vi "Ex 05 - Multiple Channels.vi"() -> ()   [LabVIEW 2026]
uses:
  Public/Data/Datatypes/MP - multi-gate inspection.ctl
  Public/Data/Datatypes/MP - multigate inspection gate parameters.ctl
  Public/Data/Datatypes/MP - hysteresis level.ctl
  Public/Data/Datatypes/MP - multigate mode.ctl
  Public/Data/Datatypes/MP - echo gate parameters.ctl
  Public/Data/Datatypes/MP - echo gate mode.ctl
  Public/Data/Datatypes/MP - data formatting.ctl
  Public/Data/Datatypes/MP - amplitude reporting mode.ctl
  Public/Data/Datatypes/MP - averaging.ctl
  Public/Data/Datatypes/MP - transmit parameters.ctl
  Public/Data/Datatypes/MP - pulser voltage.ctl
  Public/Data/Datatypes/MP - pulse damping.ctl
  Public/Data/Datatypes/MP - test parameters.ctl
  Public/Data/Datatypes/MP - receive parameters.ctl
  Public/Data/Datatypes/MP - display gate.ctl
  Public/Data/Datatypes/MP - waveform type.ctl
  Public/Data/Datatypes/MP - analogue filter.ctl
  Public/Data/Datatypes/MP - frequency filter.ctl
  Public/Data/Datatypes/MP - digital filtering.ctl
  Public/Data/Datatypes/MP - high pass filter.ctl
  Public/Data/Datatypes/MP - low pass filter.ctl
  Public/Data/Datatypes/TCP config.ctl
  Public/Data/Datatypes/MP - data output format.ctl
  Public/Data/Datatypes/MP - sample frequency.ctl
  Public/Data/Datatypes/MP - instrument type.ctl
  SubVIs/Main Program State - Enum.ctl
  <vilib>/ErrorRing/Error Ring.xnode
  MicroPulse_Driver.lvlib
panel:
  out "Instrument Type":T1
  out "Sample Frequency out":T2 caption="Sample Frequency"
  out "Stop":bool
  in  "Sample Frequency":T2
  in  "PRF":u16=500 caption="[PRF]" min=1 max=20000 step=100 format="%dHz"
  in  "Data Output Format":T3=enum."8-bit Mode" caption="[DOF]"
  in  "Gate No. 2":i32=1
  out "peak data 2":cluster{"Time":dbl[], "Level":u16[]} {"Time" format="%_6g"}
  out "A-Scan + Peaks 2":cluster{"timebase":dbl[], "data":u16[]}[](graph) caption="A-Scan + Peaks Test 2"
  out "running average PRF 2":dbl format="%0.2f"
  out "live error out 2":errorcluster
  in  "Channel Tab":enum32{"Test 1", "Test 2"}(tab)
  in  "Test 1 Tab":enum32{"Ultrasonic Parameters", "Gates"}(tab)
  in  "Data Formatting":T4={"Amplitude Mode"=enum."Peaks + Ascan for Multigate", "Averaging"=enum."None", "Coupling Level"=0} {"Coupling Level" max=4095 step=1}
  in  "Transmit Parameters":T7={"Pulse Voltage"=enum."50V", "Pulse Shape"={"Damping"=enum."660W", "Width"=250}} {"Pulse Shape"."Width" min=16 max=1010 step=50 format="%.0fns"}
  in  "Test Parameters":T10={"Test No."=1, "Tx Channel"=1, "Rx Channel"=1} {"Rx Channel" min=1 max=1024; "Tx Channel" min=1 max=1024}
  in  "Receive Parameters":T11={"Display Gate"={"Start"=0.0, "Length"=100.0}, "Delay"=0.0, "Waveform Type"=enum."Rectified Signal", "Gain"=50.0, "Analogue Filtering"={"Bandpass"=enum."No change", "Smoothing"=1}, "Digital Filtering"={"High Pass Filter"=enum."None", "Low Pass Filter"=enum."None"}} {"Delay" format="%#_g us"; "Display Gate"."Length" min=0.0 max=64000.0 step=1.0 format="%#_g us"; "Display Gate"."Start" min=0.0 max=64000.0 step=1.0 format="%#_g us"; "Analogue Filtering"."Smoothing" min=1 max=11 step=1; "Gain" min=-6.0 max=70.0 step=0.25 format="%.2fdB"}
  in  "Multi Gate Inspection":T19={"Gate 1"={"Start (us)"=15.0, "Length (us)"=10.0, "Threshold"=80, "Enabled?"=TRUE, "Max # Peaks"=8, "Hysteresis"=enum."6dB", "Mode"=enum."All Peaks In Gate", "Inverted?"=FALSE, "Colour "=16716306}, "Gate 2"={"Start (us)"=30.0, "Length (us)"=10.0, "Threshold"=50, "Enabled?"=TRUE, "Max # Peaks"=8, "Hysteresis"=enum."6dB", "Mode"=enum."All Peaks In Gate", "Inverted?"=FALSE, "Colour "=641024}, "Gate 3"={"Start (us)"=50.0, "Length (us)"=10.0, "Threshold"=30, "Enabled?"=TRUE, "Max # Peaks"=8, "Hysteresis"=enum."6dB", "Mode"=enum."All Peaks In Gate", "Inverted?"=FALSE, "Colour "=4532}, "Gate 4"={"Start (us)"=65.0, "Length (us)"=10.0, "Threshold"=10, "Enabled?"=TRUE, "Max # Peaks"=8, "Hysteresis"=enum."6dB", "Mode"=enum."All Peaks In Gate", "Inverted?"=FALSE, "Colour "=8978537}} {"Gate 4"."Max # Peaks" min=1 max=80 step=1; "Gate 4"."Threshold" min=10 step=10; "Gate 4"."Length (us)" min=0.0 max=96000.0 step=1.0; "Gate 4"."Start (us)" min=0.0 max=64000.0 step=1.0; "Gate 3"."Max # Peaks" min=1 max=80 step=1; "Gate 3"."Threshold" min=10 step=10; "Gate 3"."Length (us)" min=0.0 max=96000.0 step=1.0; "Gate 3"."Start (us)" min=0.0 max=64000.0 step=1.0; "Gate 2"."Max # Peaks" min=1 max=80 step=1; "Gate 2"."Threshold" min=10 step=10; "Gate 2"."Length (us)" min=0.0 max=96000.0 step=1.0; "Gate 2"."Start (us)" min=0.0 max=64000.0 step=1.0; "Gate 1"."Max # Peaks" min=1 max=80 step=1; "Gate 1"."Threshold" min=10 step=10; "Gate 1"."Length (us)" min=0.0 max=96000.0 step=1.0; "Gate 1"."Start (us)" min=0.0 max=64000.0 step=1.0}
  in  "Echo Gate Parameters":T23={"Start (us)"=15.0, "Length (us)"=20.0, "Threshold"=10, "Colour"=2731480} {"Threshold" min=10 max=4095 step=10; "Length (us)" min=0.0 max=96000.0 step=1.0; "Start (us)" min=0.0 max=64000.0 step=1.0}
  in  "Echo Gate Mode":T24
  in  "Test 1 Tab 2":enum32{"Ultrasonic Parameters", "Gates"}(tab)
  in  "Data Formatting 2":T4={"Amplitude Mode"=enum."Peaks + Ascan for Multigate", "Averaging"=enum."None", "Coupling Level"=0} {"Coupling Level" max=4095 step=1}
  in  "Transmit Parameters 2":T7={"Pulse Voltage"=enum."50V", "Pulse Shape"={"Damping"=enum."660W", "Width"=250}} {"Pulse Shape"."Width" min=16 max=1010 step=50 format="%.0fns"}
  in  "Test Parameters 2":T10={"Test No."=1, "Tx Channel"=2, "Rx Channel"=2} {"Rx Channel" min=1 max=1024; "Tx Channel" min=1 max=1024}
  in  "Receive Parameters 2":T11={"Display Gate"={"Start"=0.0, "Length"=100.0}, "Delay"=0.0, "Waveform Type"=enum."Rectified Signal", "Gain"=50.0, "Analogue Filtering"={"Bandpass"=enum."No change", "Smoothing"=1}, "Digital Filtering"={"High Pass Filter"=enum."None", "Low Pass Filter"=enum."None"}} {"Delay" format="%#_g us"; "Display Gate"."Length" min=0.0 max=64000.0 step=1.0 format="%#_g us"; "Display Gate"."Start" min=0.0 max=64000.0 step=1.0 format="%#_g us"; "Analogue Filtering"."Smoothing" min=1 max=11 step=1; "Gain" min=-6.0 max=70.0 step=0.25 format="%.2fdB"}
  in  "Multi Gate Inspection 2":T19={"Gate 1"={"Start (us)"=15.0, "Length (us)"=10.0, "Threshold"=80, "Enabled?"=TRUE, "Max # Peaks"=8, "Hysteresis"=enum."6dB", "Mode"=enum."All Peaks In Gate", "Inverted?"=FALSE, "Colour "=16716306}, "Gate 2"={"Start (us)"=30.0, "Length (us)"=10.0, "Threshold"=50, "Enabled?"=TRUE, "Max # Peaks"=8, "Hysteresis"=enum."6dB", "Mode"=enum."All Peaks In Gate", "Inverted?"=FALSE, "Colour "=641024}, "Gate 3"={"Start (us)"=50.0, "Length (us)"=10.0, "Threshold"=30, "Enabled?"=TRUE, "Max # Peaks"=8, "Hysteresis"=enum."6dB", "Mode"=enum."All Peaks In Gate", "Inverted?"=FALSE, "Colour "=4532}, "Gate 4"={"Start (us)"=65.0, "Length (us)"=10.0, "Threshold"=10, "Enabled?"=TRUE, "Max # Peaks"=8, "Hysteresis"=enum."6dB", "Mode"=enum."All Peaks In Gate", "Inverted?"=FALSE, "Colour "=8978537}} {"Gate 4"."Max # Peaks" min=1 max=80 step=1; "Gate 4"."Threshold" min=10 step=10; "Gate 4"."Length (us)" min=0.0 max=96000.0 step=1.0; "Gate 4"."Start (us)" min=0.0 max=64000.0 step=1.0; "Gate 3"."Max # Peaks" min=1 max=80 step=1; "Gate 3"."Threshold" min=10 step=10; "Gate 3"."Length (us)" min=0.0 max=96000.0 step=1.0; "Gate 3"."Start (us)" min=0.0 max=64000.0 step=1.0; "Gate 2"."Max # Peaks" min=1 max=80 step=1; "Gate 2"."Threshold" min=10 step=10; "Gate 2"."Length (us)" min=0.0 max=96000.0 step=1.0; "Gate 2"."Start (us)" min=0.0 max=64000.0 step=1.0; "Gate 1"."Max # Peaks" min=1 max=80 step=1; "Gate 1"."Threshold" min=10 step=10; "Gate 1"."Length (us)" min=0.0 max=96000.0 step=1.0; "Gate 1"."Start (us)" min=0.0 max=64000.0 step=1.0}
  in  "Echo Gate Parameters 2":T23={"Start (us)"=15.0, "Length (us)"=20.0, "Threshold"=10, "Colour"=2731480} {"Threshold" min=10 max=4095 step=10; "Length (us)" min=0.0 max=96000.0 step=1.0; "Start (us)" min=0.0 max=64000.0 step=1.0}
  in  "Echo Gate Mode 2":T24
  in  "Gate No.":i32=1
  out "peak data":cluster{"Time":dbl[], "Level":u16[]} {"Time" format="%_6g"}
  out "A-Scan + Peaks":cluster{"timebase":dbl[], "data":u16[]}[](graph) caption="A-Scan + Peaks Test 1"
  in  "Single Scan":bool
  in  "Stop Streaming":bool
  in  "Start Streaming":bool
  out "Command List":string
  in  "QUIT":bool
  out "running average PRF":dbl format="%0.2f"
  out "live error out":errorcluster
  out "message count":i32
  out "System Messages":string
  in  "TCP config":T25={"Connection ID"=refnum, "IP address"="10.1.1.2", "host port"=1067, "OC timeout"=5000, "Read timeout"=2000, "Write timeout"=100} {"Write timeout" format="%dms"; "Read timeout" format="%dms"; "OC timeout" format="%dms"}
  # "Example 05 - Multiple Channels\n\nSet all controls to the required values\nbefore running the VI.\n\nWhile running, test parameters may be changed."
  # "Tx and Rx Channels MUST be set BEFORE running"
  # "TEST 1"
  # "TEST 2"
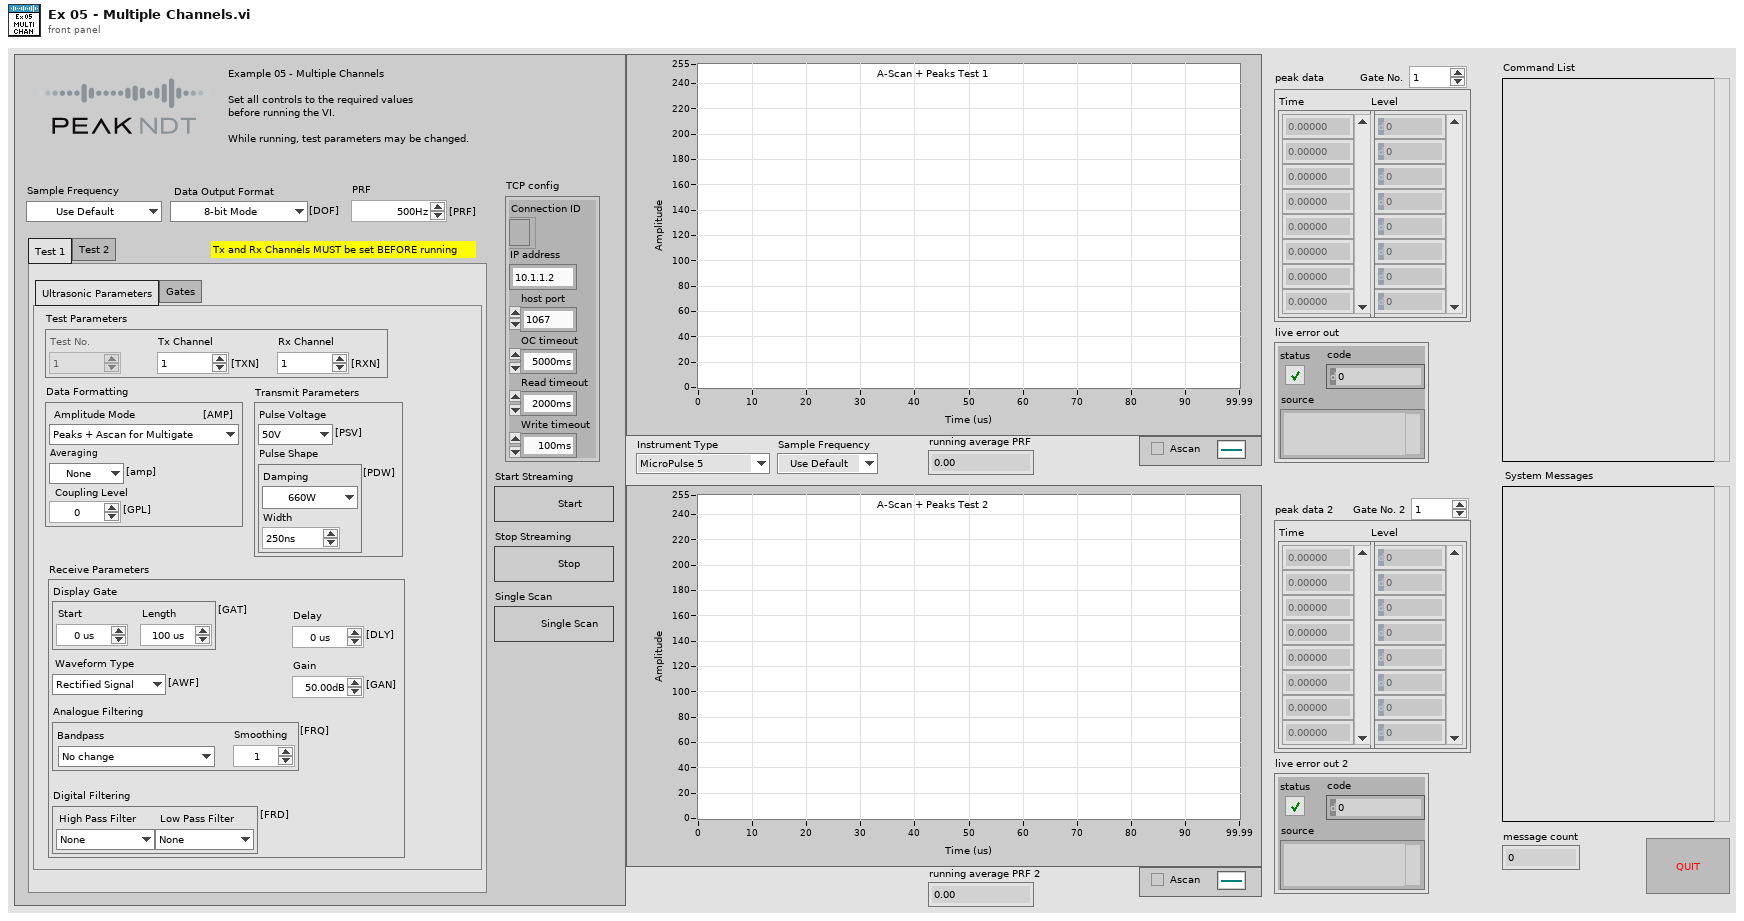
[diagram p1: front panel]
types:
  T1 = typedef "MicroPulse_Driver.lvlib/MP - instrument type.ctl" = enum16{"MicroPulse 5", "LT1", "LT2", "LTPA", "MPLT", "MicroPulse 6", "PipeScanner", "<MicroPulse>", "Micropulse 4", "Simulated Data"}
  T2 = typedef "MicroPulse_Driver.lvlib/MP - sample frequency.ctl" = enum16{"Use Default", "200MHz (LT2 only)", "100MHz", "50MHz", "25MHz", "10MHz"}
  T3 = typedef "MicroPulse_Driver.lvlib/MP - data output format.ctl" = enum16{"", "8-bit Mode", "10-bit Mode", "12-bit Mode", "16-bit Mode", "8-bit Log Mode", "12-bit Packed Mode"}
  T4 = typedef "MicroPulse_Driver.lvlib/MP - data formatting.ctl" = cluster{"Amplitude Mode":T5, "Averaging":T6, "Coupling Level":u32}
  T5 = typedef "MicroPulse_Driver.lvlib/MP - amplitude reporting mode.ctl" = enum16{"1st Peak in gate", "Maximum Peak in gate", "All Peaks", "Ascan Data", "1st Threshold Crossing Peak", "Ascan + Peaks", "All Peaks for Multigate", "Peaks + Ascan for Multigate", "Peaks + P_Ascan for Multigate", "Full Matrix Capture"}
  T6 = typedef "MicroPulse_Driver.lvlib/MP - averaging.ctl" = enum16{"None", "2", "4", "8", "16", "32", "64", "128", "256"}
  T7 = typedef "MicroPulse_Driver.lvlib/MP - transmit parameters.ctl" = cluster{"Pulse Voltage":T8, "Pulse Shape":cluster{"Damping":T9, "Width":u32}}
  T8 = typedef "MicroPulse_Driver.lvlib/MP - pulser voltage.ctl" = enum16{"50V", "100V", "150V", "200V", "250V", "300V"}
  T9 = typedef "MicroPulse_Driver.lvlib/MP - pulse damping.ctl" = enum16{"660W", "458W", "220W", "149W", "102W", "82W", "63W", "51W"}
  T10 = typedef "MicroPulse_Driver.lvlib/MP - test parameters.ctl" = cluster{"Test No.":u32, "Tx Channel":u32, "Rx Channel":u32}
  T11 = typedef "MicroPulse_Driver.lvlib/MP - receive parameters.ctl" = cluster{"Display Gate":T12, "Delay":dbl, "Waveform Type":T13, "Gain":dbl, "Analogue Filtering":T14, "Digital Filtering":T16}
  T12 = typedef "MicroPulse_Driver.lvlib/MP - display gate.ctl" = cluster{"Start":dbl, "Length":dbl}
  T13 = typedef "MicroPulse_Driver.lvlib/MP - waveform type.ctl" = enum16{"Rectified Signal", "RF Signal", "+Half Wave", "-Half Wave"}
  T14 = typedef "MicroPulse_Driver.lvlib/MP - analogue filter.ctl" = cluster{"Bandpass":T15, "Smoothing":u16}
  T15 = typedef "MicroPulse_Driver.lvlib/MP - frequency filter.ctl" = enum16{"No change", "1MHz Bandpass", "2MHz Bandpass", "4MHz Bandpass", "5MHz Bandpass", "10MHz Bandpass", "2.5-18MHz Broadband", "0.75-12MHz  Broadband", "0.5MHz Bandpass", "5MHz 2nd Order TOFD", "10MHz 2nd Order TOFD", "3.0-25MHz Broadband", "3.0-30MHz Broadband"}
  T16 = typedef "MicroPulse_Driver.lvlib/MP - digital filtering.ctl" = cluster{"High Pass Filter":T17, "Low Pass Filter":T18}
  T17 = typedef "MicroPulse_Driver.lvlib/MP - high pass filter.ctl" = enum16{"None", "0.7MHz", "1.5MHz", "4.0MHz", "7.5MHz", "10.0MHz", "User Defined"}
  T18 = typedef "MicroPulse_Driver.lvlib/MP - low pass filter.ctl" = enum16{"None", "1.8MHz", "3.0MHz", "6.0MHz", "8.0MHz", "12.0MHz", "User Defined"}
  T19 = typedef "MicroPulse_Driver.lvlib/MP - multi-gate inspection.ctl" = cluster{"Gate 1":T20, "Gate 2":T20, "Gate 3":T20, "Gate 4":T20}
  T20 = typedef "MicroPulse_Driver.lvlib/MP - multigate inspection gate parameters.ctl" = cluster{"Start (us)":dbl, "Length (us)":dbl, "Threshold":u16, "Enabled?":bool, "Max # Peaks":u16, "Hysteresis":T21, "Mode":T22, "Inverted?":bool, "Colour ":u32}
  T21 = typedef "MicroPulse_Driver.lvlib/MP - hysteresis level.ctl" = enum16{"None", "3dB", "6dB", "9dB", "12dB"}
  T22 = typedef "MicroPulse_Driver.lvlib/MP - multigate mode.ctl" = enum16{"1st Peak in Gate", "Largest Peak In Gate", "All Peaks In Gate", "1st Threshold Crossing"}
  T23 = typedef "MicroPulse_Driver.lvlib/MP - echo gate parameters.ctl" = cluster{"Start (us)":dbl, "Length (us)":dbl, "Threshold":u16, "Colour":u32}
  T24 = typedef "MicroPulse_Driver.lvlib/MP - echo gate mode.ctl" = enum16{"Echo Trigger OFF", "Echo Gate Display Mode", "Echo Trigger ON", "Multi Gate or FMC Mode", "Reserved", "PA - Echo Trigger ON"}
  T25 = typedef "MicroPulse_Driver.lvlib/TCP config.ctl" = cluster{"Connection ID":refnum<k5>, "IP address":string, "host port":u16, "OC timeout":i32, "Read timeout":i32, "Write timeout":i32}
  T26 = typedef "Main Program State - Enum.ctl" = enum16{"Initialise", "Init HW", "Run", "Reset HW", "Shutdown"}
  T27 = typedef "MicroPulse_Driver.lvlib/MP-Registry Data-Cluster.ctl" = cluster{"Instrument Type":T1, "Serial #":u64, "Sample Frequency":T2, "dt (us)":dbl, "DOF":T3, "Material Velocity":dbl, "Asynch Reads":T28, "NUM of Tests":u32, "System Details":T29, "Gates":T31[], "Encoders":T32[], "CMD LUT":variant, "Command List":string}
  T28 = typedef "MicroPulse_Driver.lvlib/MP - asynch read mode.ctl" = enum16{"Disabled", "Enabled"}
  T29 = typedef "MicroPulse_Driver.lvlib/MP - general system status.ctl" = cluster{"System Type":T1, "Serial No.":u64, "Channels":cluster{"Conv":u8, "PA":u16, "Extra":u32}, "Sample Frequency":cluster{"Default":u8, "Actual":u8}, "Software Versions":string, "Data Output Format":cluster{"Default":T3, "Actual":T3}, "Temperatures":cluster{"System":u8, "Processor":u8, "Slave Sys":u8, "Slave Proc":u8}, "Tx Buffer Size":u32, "System Error":string, "No. of Cards":u8, "DAC Gain":i16, "Uptimes":cluster{"since Power":u32, "since RSTS":u32, "since SRST":u32}, "Voltages":cluster{"Nominal":dbl, "Measured":dbl, "Difference":dbl}[], "Interface Cards":T30[]}
  T30 = typedef "MicroPulse_Driver.lvlib/MP - interface card status.ctl" = cluster{"Status":u8, "Map":u8, "Board - T":u8, "FPGA - T":u8, "PAIF Status":string, "Version":string}
  T31 = typedef "MicroPulse_Driver.lvlib/MP - Registry Gates.ctl" = cluster{"Display Gate":T12, "ETM Mode":T24, "Echo Gate":T23, "Insp Gates":T20[]}
  T32 = typedef "MicroPulse_Driver.lvlib/MP - encoder settings.ctl" = cluster{"Encoder Type":T33, "Counts/mm":u32, "Enable Termination?":bool, "Multiplier":u32, "Backlash Period (s)":dbl, "Encoder Filter":u32}
  T33 = typedef "MicroPulse_Driver.lvlib/MP - encoder type.ctl" = enum16{"Quadrature", "Step/Direction"}
  T34 = typedef "MicroPulse_Driver.lvlib/MP - scan data info.ctl" = cluster{"Message Header":u16, "Error Message":u16, "Test No.":u32, "Channel No.":u8, "Sweep No.":u32, "Gate No.":u32, "DOF":T3, "retain data":T35, "scan data":u16[], "scan length":i32, "scan index":i32, "peak data":cluster{"timebase":u16[], "data":u16[]}, "#peaks":i32, "PRF":dbl, "IP":cluster{"Axis No.":u8, "Location":u32, "MIP location":u32, "MIP?":bool}, "echo range":u16, "ETG":bool, "CAL 0 complete":bool, "Axis Positions":T36}
  T35 = typedef "MicroPulse_Driver.lvlib/MP - retain scan.ctl" = enum16{"None", "Ascan", "Peaks"}
  T36 = typedef "MicroPulse_Driver.lvlib/MP - axis positions (LLC).ctl" = cluster{"Axis 1":u32, "Axis 2":u32, "Axis 3":u32, "Axis 4":u32, "Status":u8}
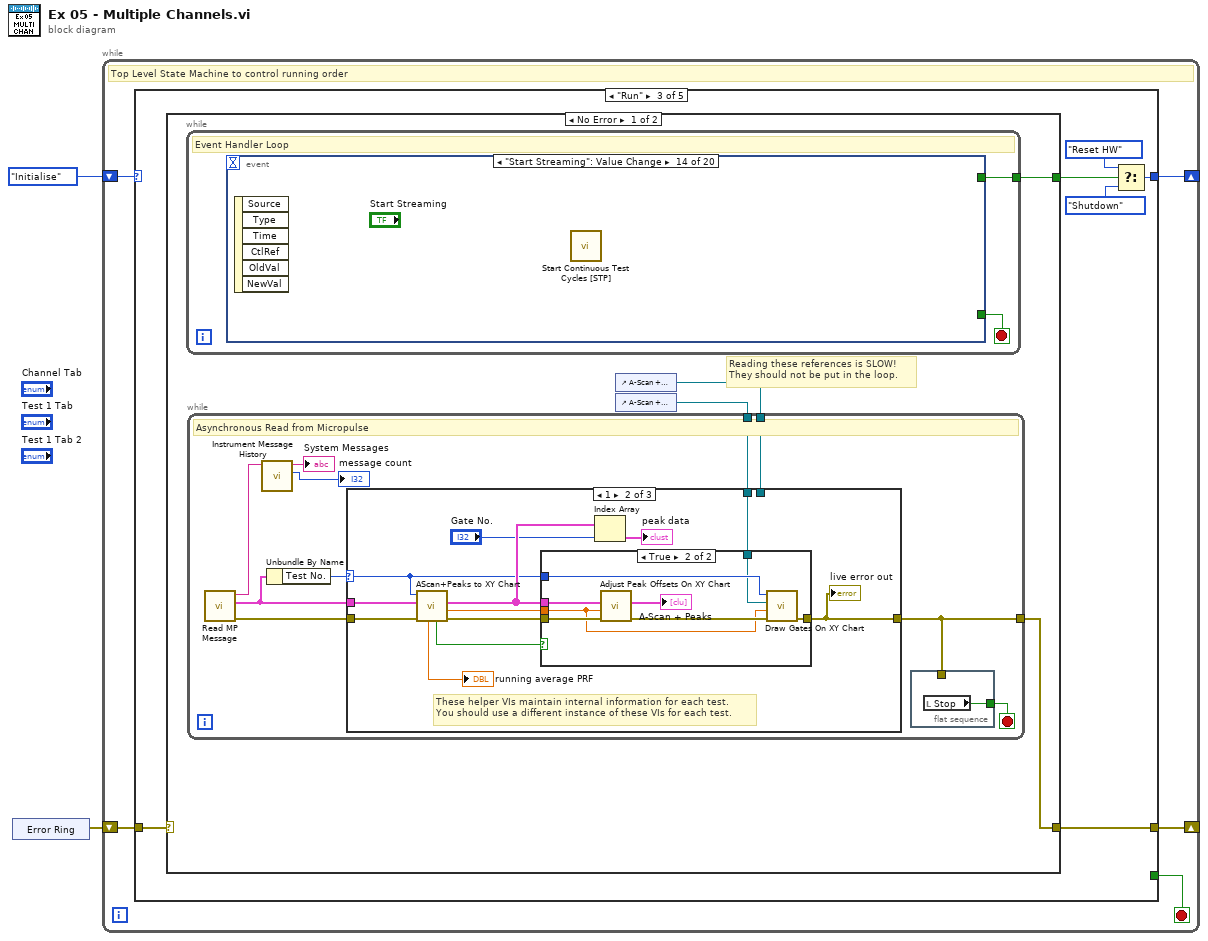
[diagram p0: block diagram]
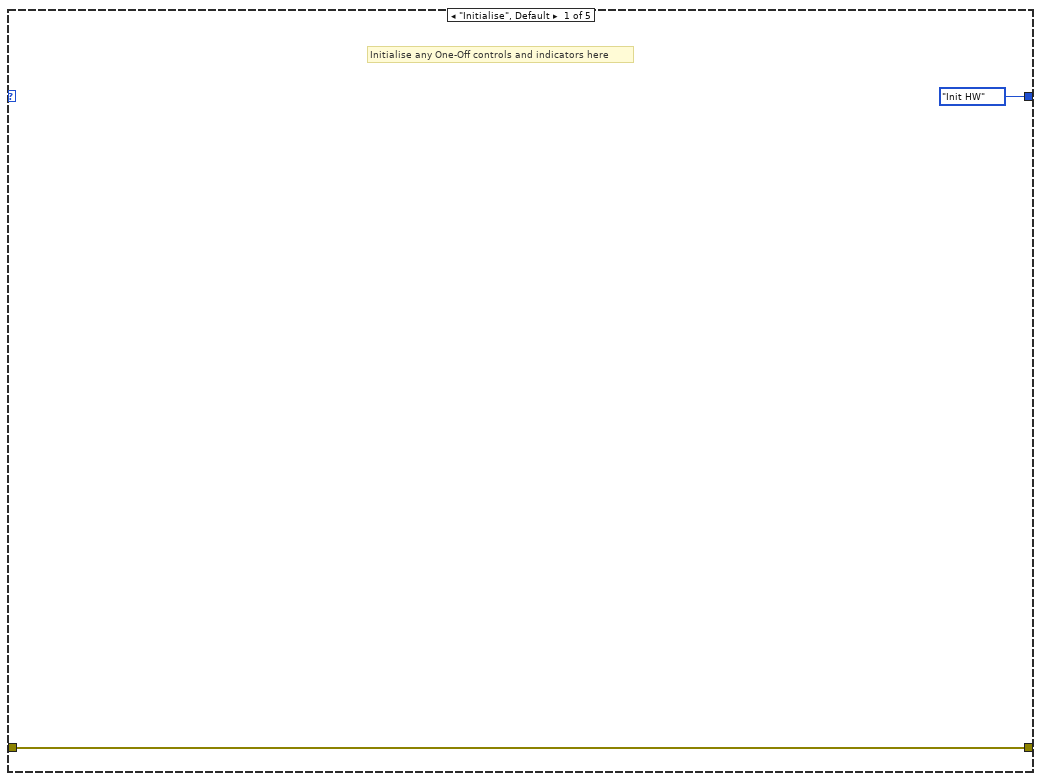
[diagram p2: hidden frame]
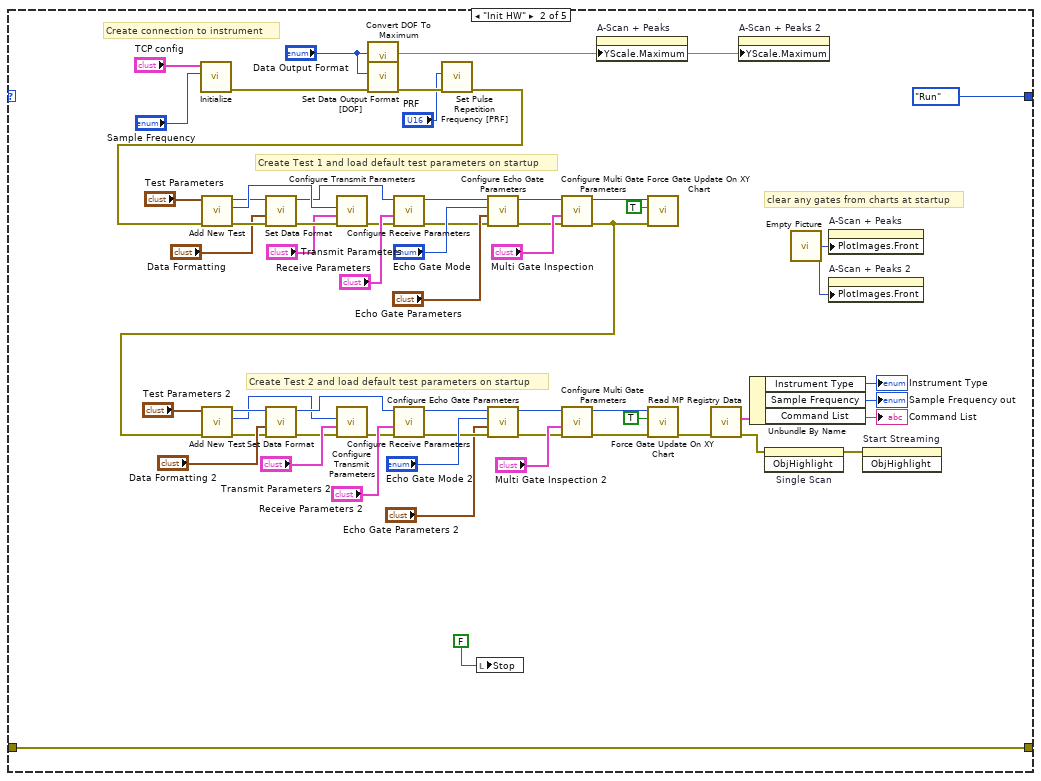
[diagram p3: hidden frame]
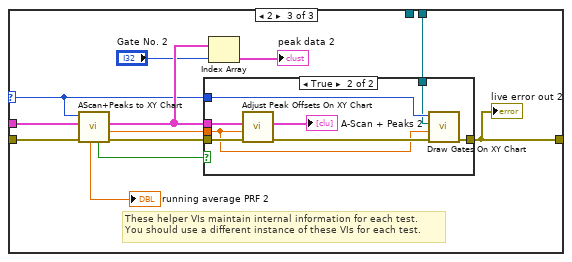
[diagram p6: hidden frame]
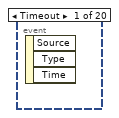
[diagram p8: hidden frame]
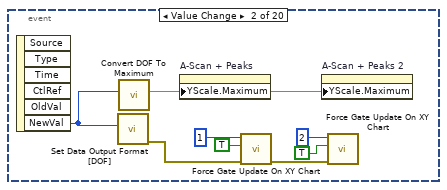
[diagram p9: hidden frame]
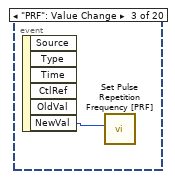
[diagram p10: hidden frame]
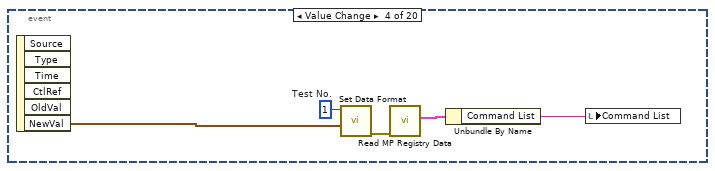
[diagram p11: hidden frame]
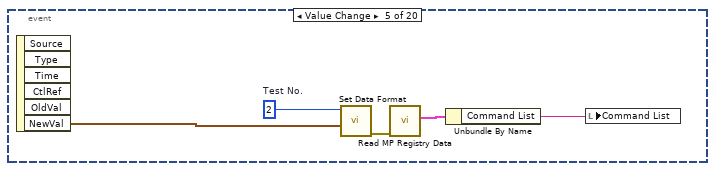
[diagram p12: hidden frame]
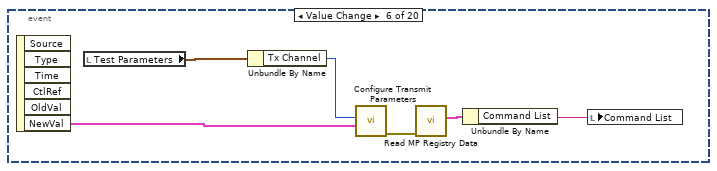
[diagram p13: hidden frame]
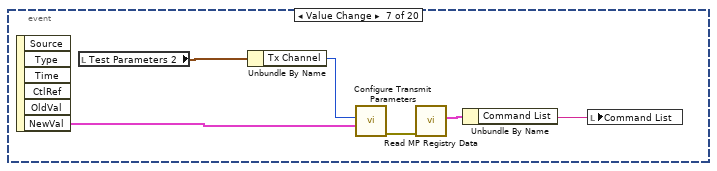
[diagram p14: hidden frame]
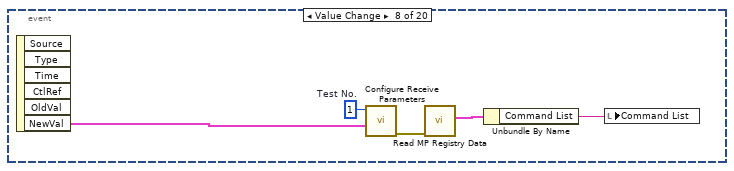
[diagram p15: hidden frame]
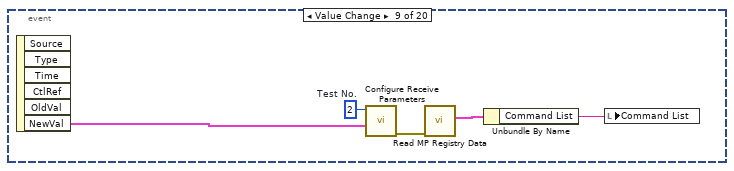
[diagram p16: hidden frame]
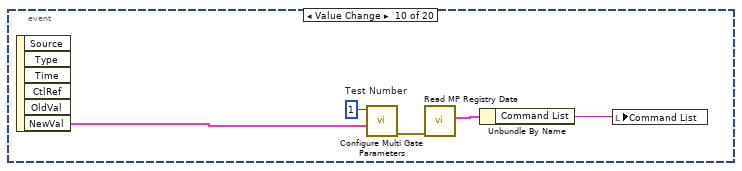
[diagram p17: hidden frame]
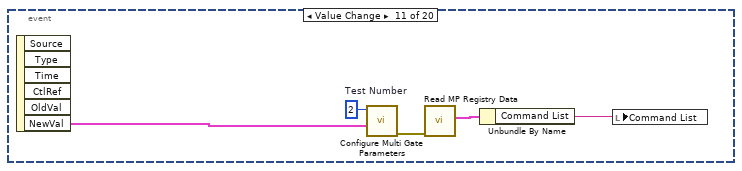
[diagram p18: hidden frame]
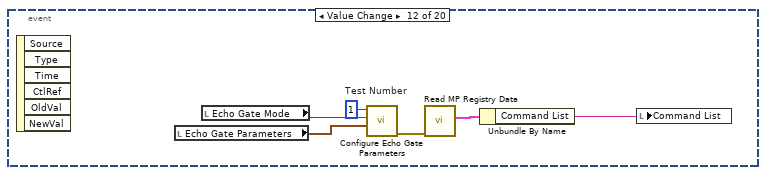
[diagram p19: hidden frame]
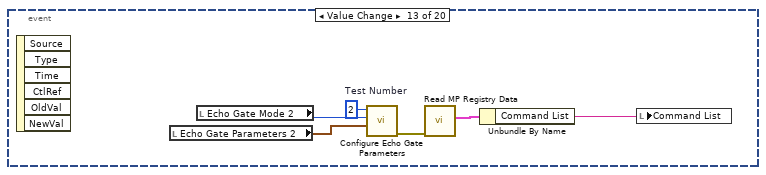
[diagram p20: hidden frame]
diagram:
  n1 = xnode "Error Ring"() -> ("error out"=w2:errorcluster)
  n2 = while {
    shift-right: [w4] -> _
    shift-left: Main_Program_State_-_Enum."Initialise" -> [w7]
    shift-right: [w5] -> _
    shift-left: w2 -> [w6]
    stop <- w3 stop-if-true
    # "Top Level State Machine to control running order"
    n3 = case shown="\"Run\"" w7 {
      tunnel: w6 -> [w8 w29 w74 w209 w214]
      tunnel: [w8 w29 w73 w208 w214] -> w5
      tunnel: [Main_Program_State_-_Enum."Init HW" Main_Program_State_-_Enum."Run" w69 Main_Program_State_-_Enum."Init HW" Main_Program_State_-_Enum."Initialise"] -> w4
      tunnel: [_ _ _ _ TRUE] -> w3
      frame "Initialise", Default {
        # "Initialise any One-Off controls and indicators here"
      }
      frame "Init HW" {
        # "Create connection to instrument"
        # "Create Test 2 and load default test parameters on startup"
        # "clear any gates from charts at startup"
        # "Create Test 1 and load default test parameters on startup"
        n4 = call "Initialize.vi"("Sample Frequency"="Sample Frequency", "TCP config"="TCP config") -> ("error out"=w15:errorcluster)  [unwired: 8 in, 1 out]
        n5 = call "Convert DOF To Maximum.vi"("Data Output Format"="Data Output Format") -> ("Data Maximum"=w12:dbl)  [unwired: 10 in]
        n6 = call "Set Data Output Format [DOF].vi"("error in (no error)"=w15, "Mode"="Data Output Format") -> ("error out"=w17:errorcluster)  [unwired: 8 in, 1 out]
        n7 = call "Set Pulse Repetition Frequency [PRF].vi"("error in (no error)"=w17, "Frequency (Hz)"="PRF") -> ("error out"=w14:errorcluster)  [unwired: 8 in, 1 out]
        n8 = call "Add New Test.vi"("error in (no error)"=w14, "Test Parameters"="Test Parameters") -> ("error out"=w45:errorcluster, "Tx Channel out"=w44:u32, "Test No. out"=w40:u32)  [unwired: 6 in, 1 out]
        n9 = call "Set Data Format.vi"("error in (no error)"=w45, "Data Formatting"="Data Formatting", "Test No."=w40) -> ("error out"=w35:errorcluster, "Test No. out"=w42:u32)  [unwired: 6 in, 1 out]
        n10 = call "Configure Transmit Parameters.vi"("error in (no error)"=w35, "Transmit Parameters"="Transmit Parameters", "Tx Channel"=w44) -> ("error out"=w34:errorcluster)  [unwired: 7 in, 1 out]
        n11 = call "Configure Receive Parameters.vi"("error in (no error)"=w34, "Receive Parameters"="Receive Parameters", "Test No."=w42) -> ("error out"=w36:errorcluster, "Test No. out"=w41:u32)  [unwired: 6 in, 1 out]
        n12 = local write "Stop"(FALSE ("stop")) -> ()
        n13 = call "Configure Echo Gate Parameters.vi"("error in (no error)"=w36, "Echo Gate Parameters"="Echo Gate Parameters", "Echo Trigger Mode"="Echo Gate Mode", "Test Number"=w41) -> ("error out"=w38:errorcluster, "Test Number Out"=w43:u32)  [unwired: 5 in, 1 out]
        n14 = call "Configure Multi Gate Parameters.vi"("error in (no error)"=w38, "Multi Gate Inspection"="Multi Gate Inspection", "Test Number"=w43) -> ("error out"=w27:errorcluster, "Test Number out"=w26:u32)  [unwired: 6 in, 1 out]
        n15 = call "Add New Test.vi"("error in (no error)"=w27, "Test Parameters"="Test Parameters 2") -> ("error out"=w59:errorcluster, "Tx Channel out"=w53:u32, "Test No. out"=w57:u32)  [unwired: 6 in, 1 out]
        n16 = call "Set Data Format.vi"("error in (no error)"=w59, "Data Formatting"="Data Formatting 2", "Test No."=w57) -> ("error out"=w60:errorcluster, "Test No. out"=w55:u32)  [unwired: 6 in, 1 out]
        n17 = call "Configure Transmit Parameters.vi"("error in (no error)"=w60, "Transmit Parameters"="Transmit Parameters 2", "Tx Channel"=w53) -> ("error out"=w61:errorcluster)  [unwired: 7 in, 1 out]
        n18 = call "Configure Receive Parameters.vi"("error in (no error)"=w61, "Receive Parameters"="Receive Parameters 2", "Test No."=w55) -> ("error out"=w62:errorcluster, "Test No. out"=w56:u32)  [unwired: 6 in, 1 out]
        n19 = call "Configure Echo Gate Parameters.vi"("error in (no error)"=w62, "Echo Gate Parameters"="Echo Gate Parameters 2", "Echo Trigger Mode"="Echo Gate Mode 2", "Test Number"=w56) -> ("error out"=w63:errorcluster, "Test Number Out"=w54:u32)  [unwired: 5 in, 1 out]
        n20 = call "Configure Multi Gate Parameters.vi"("error in (no error)"=w63, "Multi Gate Inspection"="Multi Gate Inspection 2", "Test Number"=w54) -> ("error out"=w24:errorcluster, "Test Number out"=w21:u32)  [unwired: 6 in, 1 out]
        n21 = property on="A-Scan + Peaks" class="XYGraph (strict)"("YScale.Maximum"=w12) -> ()  [unwired: 2 in, 2 out]
        n22 = call "Force Gate Update On XY Chart.vi"("error in (no error)"=w27, "Set?"=TRUE, "Test No."=w26) -> ()  [unwired: 6 in, 3 out]
        n23 = call "Force Gate Update On XY Chart.vi"("error in (no error)"=w24, "Set?"=TRUE, "Test No."=w21) -> ("error out"=w23:errorcluster)  [unwired: 6 in, 2 out]
        n24 = call "Read MP Registry Data.vi"("error in (no error)"=w23) -> ("error out"=w51:errorcluster, "Micropulse Data"=w49:T27)  [unwired: 7 in, 2 out]
        n25 = property on="A-Scan + Peaks 2" class="XYGraph (strict)"("YScale.Maximum"=w12) -> ()  [unwired: 2 in, 2 out]
        n26 = Unbundle By Name(w49) -> ("Instrument Type"=→"Instrument Type":T1, "Sample Frequency"=→"Sample Frequency out":T2, "Command List"=→"Command List":string)
        n27 = invoke on="Single Scan" class="Bool" method="ObjHighlight"(error in=w51) -> (error out=w52:errorcluster)  [unwired: 2 in, 2 out]
        n28 = call "Empty Picture"() -> ("empty picture"=w28:picture)
        n29 = property on="A-Scan + Peaks" class="XYGraph (strict)"("PlotImages.Front"=w28) -> ()  [unwired: 2 in, 2 out]
        n30 = property on="A-Scan + Peaks 2" class="XYGraph (strict)"("PlotImages.Front"=w28) -> ()  [unwired: 2 in, 2 out]
        n31 = invoke on="Start Streaming" class="Bool" method="ObjHighlight"(error in=w52) -> ()  [unwired: 2 in, 3 out]
      }
      frame "Run" {
        n32 = case shown="No Error" w74 {
          selector: w74 -> [_ w207]
          tunnel: [w76 w207] -> w73
          tunnel: [w75 _] -> w70
          frame No Error {
            # "Reading these references is SLOW!\nThey should not be put in the loop."
            n33 = while {
              tunnel: [w133] -> w75
              stop <- w134 stop-if-true
              # "Event Handler Loop"
              n34 = event shown="[13] \"Start Streaming\": Value Change" {
                selector: _ -> [_ _ _ _ _ _ _ _ _ _ _ _ _ _ _ _ _ _ _ _]
                dyn-events: _ -> [_ _ _ _ _ _ _ _ _ _ _ _ _ _ _ _ _ _ _ _]
                timeout: _ -> [_ _ _ _ _ _ _ _ _ _ _ _ _ _ _ _ _ _ _ _]
                tunnel: [_ _ _ _ _ _ _ _ _ _ _ _ _ _ _ _ _ _ w203 TRUE ("stop")] -> w134
                tunnel: [_ _ _ _ _ _ _ _ _ _ _ _ _ _ _ _ _ _ TRUE _] -> w133
                event Timeout {
                  n35 = event-data() -> ()  [unwired: 1 in, 3 out]
                }
                event Value Change {
                  n36 = event-data() -> ("NewVal"=w136:T3)  [unwired: 1 in, 5 out]
                  n37 = call "Set Data Output Format [DOF].vi"("Mode"=w136) -> ("error out"=w138:errorcluster)  [unwired: 9 in, 1 out]
                  n38 = call "Convert DOF To Maximum.vi"("Data Output Format"=w136) -> ("Data Maximum"=w135:dbl)  [unwired: 10 in]
                  n39 = property on="A-Scan + Peaks" class="XYGraph (strict)"("YScale.Maximum"=w135) -> ()  [unwired: 2 in, 2 out]
                  n40 = call "Force Gate Update On XY Chart.vi"("error in (no error)"=w138, "Set?"=TRUE, "Test No."=u32 1) -> ("error out"=w137:errorcluster)  [unwired: 6 in, 2 out]
                  n41 = property on="A-Scan + Peaks 2" class="XYGraph (strict)"("YScale.Maximum"=w135) -> ()  [unwired: 2 in, 2 out]
                  n42 = call "Force Gate Update On XY Chart.vi"("error in (no error)"=w137, "Set?"=TRUE, "Test No."=u32 2) -> ()  [unwired: 6 in, 3 out]
                }
                event "PRF": Value Change {
                  n43 = event-data() -> ("NewVal"=w143:u16)  [unwired: 1 in, 5 out]
                  n44 = call "Set Pulse Repetition Frequency [PRF].vi"("Frequency (Hz)"=w143) -> ()  [unwired: 9 in, 2 out]
                }
                event Value Change {
                  w145 = u32 1  # Test No.
                  n45 = event-data() -> ("NewVal"=w144:T4)  [unwired: 1 in, 5 out]
                  n46 = call "Set Data Format.vi"("Data Formatting"=w144, "Test No."=w145) -> ("error out"=w148:errorcluster)  [unwired: 7 in, 2 out]
                  n47 = call "Read MP Registry Data.vi"("error in (no error)"=w148) -> ("Micropulse Data"=w147:T27)  [unwired: 7 in, 3 out]
                  n48 = Unbundle By Name(w147) -> ("Command List"=w146:string)
                  n49 = local write "Command List"(w146) -> ()
                }
                event Value Change {
                  w150 = u32 2  # Test No.
                  n50 = event-data() -> ("NewVal"=w149:T4)  [unwired: 1 in, 5 out]
                  n51 = call "Set Data Format.vi"("Data Formatting"=w149, "Test No."=w150) -> ("error out"=w153:errorcluster)  [unwired: 7 in, 2 out]
                  n52 = call "Read MP Registry Data.vi"("error in (no error)"=w153) -> ("Micropulse Data"=w152:T27)  [unwired: 7 in, 3 out]
                  n53 = Unbundle By Name(w152) -> ("Command List"=w151:string)
                  n54 = local write "Command List"(w151) -> ()
                }
                event Value Change {
                  n55 = event-data() -> ("NewVal"=w158:T7)  [unwired: 1 in, 5 out]
                  n56 = local read "Test Parameters"() -> (w159:T10)
                  n57 = Unbundle By Name(w159) -> ("Tx Channel"=w157:u32)
                  n58 = call "Configure Transmit Parameters.vi"("Transmit Parameters"=w158, "Tx Channel"=w157) -> ("error out"=w155:errorcluster)  [unwired: 8 in, 1 out]
                  n59 = call "Read MP Registry Data.vi"("error in (no error)"=w155) -> ("Micropulse Data"=w156:T27)  [unwired: 7 in, 3 out]
                  n60 = Unbundle By Name(w156) -> ("Command List"=w154:string)
                  n61 = local write "Command List"(w154) -> ()
                }
                event Value Change {
                  n62 = event-data() -> ("NewVal"=w164:T7)  [unwired: 1 in, 5 out]
                  n63 = local read "Test Parameters 2"() -> (w165:T10)
                  n64 = Unbundle By Name(w165) -> ("Tx Channel"=w163:u32)
                  n65 = call "Configure Transmit Parameters.vi"("Transmit Parameters"=w164, "Tx Channel"=w163) -> ("error out"=w161:errorcluster)  [unwired: 8 in, 1 out]
                  n66 = call "Read MP Registry Data.vi"("error in (no error)"=w161) -> ("Micropulse Data"=w162:T27)  [unwired: 7 in, 3 out]
                  n67 = Unbundle By Name(w162) -> ("Command List"=w160:string)
                  n68 = local write "Command List"(w160) -> ()
                }
                event Value Change {
                  w166 = u32 1  # Test No.
                  n69 = event-data() -> ("NewVal"=w170:T11)  [unwired: 1 in, 5 out]
                  n70 = call "Configure Receive Parameters.vi"("Receive Parameters"=w170, "Test No."=w166) -> ("error out"=w169:errorcluster)  [unwired: 7 in, 2 out]
                  n71 = call "Read MP Registry Data.vi"("error in (no error)"=w169) -> ("Micropulse Data"=w167:T27)  [unwired: 7 in, 3 out]
                  n72 = Unbundle By Name(w167) -> ("Command List"=w168:string)
                  n73 = local write "Command List"(w168) -> ()
                }
                event Value Change {
                  w171 = u32 2  # Test No.
                  n74 = event-data() -> ("NewVal"=w175:T11)  [unwired: 1 in, 5 out]
                  n75 = call "Configure Receive Parameters.vi"("Receive Parameters"=w175, "Test No."=w171) -> ("error out"=w174:errorcluster)  [unwired: 7 in, 2 out]
                  n76 = call "Read MP Registry Data.vi"("error in (no error)"=w174) -> ("Micropulse Data"=w172:T27)  [unwired: 7 in, 3 out]
                  n77 = Unbundle By Name(w172) -> ("Command List"=w173:string)
                  n78 = local write "Command List"(w173) -> ()
                }
                event Value Change {
                  w176 = u32 1  # Test Number
                  n79 = event-data() -> ("NewVal"=w180:T19)  [unwired: 1 in, 5 out]
                  n80 = call "Configure Multi Gate Parameters.vi"("Multi Gate Inspection"=w180, "Test Number"=w176) -> ("error out"=w179:errorcluster)  [unwired: 7 in, 2 out]
                  n81 = call "Read MP Registry Data.vi"("error in (no error)"=w179) -> ("Micropulse Data"=w178:T27)  [unwired: 7 in, 3 out]
                  n82 = Unbundle By Name(w178) -> ("Command List"=w177:string)
                  n83 = local write "Command List"(w177) -> ()
                }
                event Value Change {
                  w181 = u32 2  # Test Number
                  n84 = event-data() -> ("NewVal"=w185:T19)  [unwired: 1 in, 5 out]
                  n85 = call "Configure Multi Gate Parameters.vi"("Multi Gate Inspection"=w185, "Test Number"=w181) -> ("error out"=w184:errorcluster)  [unwired: 7 in, 2 out]
                  n86 = call "Read MP Registry Data.vi"("error in (no error)"=w184) -> ("Micropulse Data"=w183:T27)  [unwired: 7 in, 3 out]
                  n87 = Unbundle By Name(w183) -> ("Command List"=w182:string)
                  n88 = local write "Command List"(w182) -> ()
                }
                event Value Change {
                  w186 = u32 1  # Test Number
                  n89 = event-data() -> ()  [unwired: 1 in, 6 out]
                  n90 = local read "Echo Gate Parameters"() -> (w189:T23)
                  n91 = local read "Echo Gate Mode"() -> (w190:T24)
                  n92 = call "Configure Echo Gate Parameters.vi"("Echo Gate Parameters"=w189, "Echo Trigger Mode"=w190, "Test Number"=w186) -> ("error out"=w191:errorcluster)  [unwired: 6 in, 2 out]
                  n93 = call "Read MP Registry Data.vi"("error in (no error)"=w191) -> ("Micropulse Data"=w188:T27)  [unwired: 7 in, 3 out]
                  n94 = Unbundle By Name(w188) -> ("Command List"=w187:string)
                  n95 = local write "Command List"(w187) -> ()
                }
                event Value Change {
                  w192 = u32 2  # Test Number
                  n96 = event-data() -> ()  [unwired: 1 in, 6 out]
                  n97 = local read "Echo Gate Parameters 2"() -> (w195:T23)
                  n98 = local read "Echo Gate Mode 2"() -> (w196:T24)
                  n99 = call "Configure Echo Gate Parameters.vi"("Echo Gate Parameters"=w195, "Echo Trigger Mode"=w196, "Test Number"=w192) -> ("error out"=w197:errorcluster)  [unwired: 6 in, 2 out]
                  n100 = call "Read MP Registry Data.vi"("error in (no error)"=w197) -> ("Micropulse Data"=w194:T27)  [unwired: 7 in, 3 out]
                  n101 = Unbundle By Name(w194) -> ("Command List"=w193:string)
                  n102 = local write "Command List"(w193) -> ()
                }
                event "Start Streaming": Value Change {
                  n103 = event-data() -> ()  [unwired: 1 in, 6 out]
                  n104 = call "Start Continuous Test Cycles [STP].vi"() -> ()  [unwired: 10 in, 2 out]
                }
                event "Stop Streaming": Value Change {
                  w198 = TRUE  # Erase All? (def F)
                  n105 = event-data() -> ()  [unwired: 1 in, 6 out]
                  n106 = call "Enter Idle Mode [STX].vi"("Erase All? (def T)"=w198) -> ()  [unwired: 9 in, 2 out]
                }
                event "Single Scan": Value Change {
                  n107 = event-data() -> ()  [unwired: 1 in, 6 out]
                  n108 = call "Start 1 Test Cycle [CAL].vi"() -> ()  [unwired: 10 in, 2 out]
                }
                event "A-Scan + Peaks": Scale Range Change {
                  n109 = event-data() -> ()  [unwired: 1 in, 8 out]
                  n110 = call "Force Gate Update On XY Chart.vi"("Set?"=TRUE, "Test No."=u32 1) -> ()  [unwired: 7 in, 3 out]
                }
                event "A-Scan + Peaks 2": Scale Range Change {
                  n111 = event-data() -> ()  [unwired: 1 in, 8 out]
                  n112 = call "Force Gate Update On XY Chart.vi"("Set?"=TRUE, "Test No."=u32 2) -> ()  [unwired: 7 in, 3 out]
                }
                event Value Change {
                  w203 = TRUE
                  # "Stop all activity and reset the hardware to change the sampling frequency"
                  n113 = event-data() -> ()  [unwired: 1 in, 6 out]
                  n114 = local write "Stop"(w203) -> ()
                }
                event "QUIT": Value Change {
                  # "set flag to stop acquisition loop"
                  n115 = event-data() -> ()  [unwired: 1 in, 6 out]
                  "Stop" <- TRUE ("Stop")
                }
              }
            }
            n116 = control-ref of="A-Scan + Peaks 2"() -> (w78:refnum<vi>)
            n117 = control-ref of="A-Scan + Peaks"() -> (w77:refnum<vi>)
            n118 = while {
              tunnel: w78 -> [w82]
              tunnel: w77 -> [w81]
              tunnel: [w80] -> w76
              stop <- w79 stop-if-true
              # "Asynchronous Read from Micropulse"
              n119 = call "Read MP Message.vi"() -> ("error out"=w83:errorcluster, "scan data info"=w84:T34, "Instrument Message"=w87:string)  [unwired: 7 in, 2 out]
              n120 = call "Instrument Message History.vi"("Instrument Message"=w87) -> ("Message Count"=→"message count":i32, "Message History out"=→"System Messages":string)  [unwired: 9 in]
              n121 = Unbundle By Name(w84) -> ("Test No."=w85:u32)
              n122 = case shown="1" w85 {
                selector: w85 -> [_ w96 w117]
                tunnel: w84 -> [_ w98 w121]
                tunnel: w83 -> [w90 w97 w120]
                tunnel: w82 -> [_ _ w114]
                tunnel: w81 -> [_ w95 _]
                tunnel: [w90 w92 w116] -> w80
                frame -1, Default {
                }
                frame 1 {
                  # "These helper VIs maintain internal information for each test.\nYou should use a different instance of these VIs for each test."
                  n123 = call "AScan+Peaks to XY Chart.vi"("error in (no error)"=w97, "scan data info"=w98, "Test No."=w96) -> ("error out"=w99:errorcluster, "Echo Range (us)"=w94:dbl, "AScan+Peaks"=w102:cluster{"timebase":dbl[], "data":u16[]}[], "Update Indicators?"=w91:bool, "Running Average PRF"=→"running average PRF":dbl)  [unwired: 3 in, 1 out]
                  n124 = case shown="True" w91 {
                    tunnel: w102 -> [_ w110]
                    tunnel: w99 -> [w103 w108]
                    tunnel: w96 -> [_ w106]
                    tunnel: w95 -> [_ w105]
                    tunnel: w94 -> [_ w104]
                    tunnel: [w103 w107] -> w92
                    frame False {
                    }
                    frame True {
                      n125 = call "Adjust Peak Offsets On XY Chart.vi"("error in (no error)"=w108, "Echo Range in"=w104, "AScan+Peaks in"=w110) -> ("error out"=w109:errorcluster, "AScan+Peaks out"=→"A-Scan + Peaks":cluster{"timebase":dbl[], "data":u16[]}[])  [unwired: 7 in]
                      n126 = call "Draw Gates On XY Chart.vi"("error in (no error)"=w109, "Echo Range"=w104, "XYGraph in"=w105, "Test No."=w106) -> ("error out"=w107:errorcluster)  [unwired: 7 in]
                    }
                  }
                  "live error out" <- w92
                  n127 = Index Array(array=w102, index="Gate No.") -> (element=→"peak data":cluster{"timebase":dbl[], "data":u16[]})
                }
                frame 2 {
                  # "These helper VIs maintain internal information for each test.\nYou should use a different instance of these VIs for each test."
                  n128 = call "AScan+Peaks to XY Chart.vi"("error in (no error)"=w120, "scan data info"=w121, "Test No."=w117) -> ("error out"=w122:errorcluster, "Echo Range (us)"=w115:dbl, "AScan+Peaks"=w123:cluster{"timebase":dbl[], "data":u16[]}[], "Update Indicators?"=w113:bool, "Running Average PRF"=→"running average PRF 2":dbl)  [unwired: 3 in, 1 out]
                  n129 = case shown="True" w113 {
                    tunnel: w123 -> [_ w132]
                    tunnel: w122 -> [w124 w130]
                    tunnel: w117 -> [_ w128]
                    tunnel: [w124 w127] -> w116
                    tunnel: w115 -> [_ w126]
                    tunnel: w114 -> [_ w125]
                    frame False {
                    }
                    frame True {
                      n130 = call "Adjust Peak Offsets On XY Chart.vi"("error in (no error)"=w130, "Echo Range in"=w126, "AScan+Peaks in"=w132) -> ("error out"=w131:errorcluster, "AScan+Peaks out"=→"A-Scan + Peaks 2":cluster{"timebase":dbl[], "data":u16[]}[])  [unwired: 7 in]
                      n131 = call "Draw Gates On XY Chart.vi"("error in (no error)"=w131, "Echo Range"=w126, "XYGraph in"=w125, "Test No."=w128) -> ("error out"=w127:errorcluster)  [unwired: 7 in]
                    }
                  }
                  "live error out 2" <- w116
                  n132 = Index Array(array=w123, index="Gate No. 2") -> (element=→"peak data 2":cluster{"timebase":dbl[], "data":u16[]})
                }
              }
              n133 = flat-sequence {
                tunnel: [w89] -> w79
                tunnel: w80 -> [_]
                frame #0 {
                  n134 = local read "Stop"() -> (w89:bool)
                }
              }
            }
          }
          frame Error {
          }
        }
        n135 = Select(t=Main_Program_State_-_Enum."Reset HW", s=w70, f=Main_Program_State_-_Enum."Shutdown") -> (s? t:f=w69:T26)
      }
      frame "Reset HW" {
        # "Close the connection to allow for reopening in the \"Init HW\" case"
        n136 = call "Close.vi"("error in (no error)"=w209) -> ("error out"=w208:errorcluster)  [unwired: 9 in, 1 out]
      }
      frame "Shutdown" {
        # "Terminate the TCP/IP connection"
        n137 = local write "Stop"(FALSE ("stop")) -> ()
        n138 = call "Close.vi"() -> ()  [unwired: 10 in, 2 out]
      }
    }
  }
